vi "CPP_HalveFirstAndLast.vi"(3 "InputArray":dbl[](array[numeric])) -> (1 "HalvedEnds":dbl[](array[numeric]))   [LabVIEW 2010]
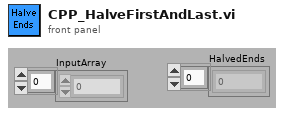
[diagram p1: front panel]
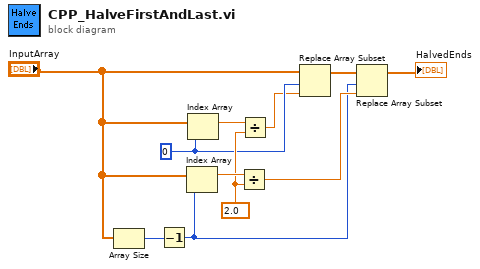
[diagram p0: block diagram]
diagram:
  w7 = 0
  w8 = 2.0
  n1 = Array Size(array="InputArray") -> (size(s)=w3:i32)
  n2 = Decrement(x=w3) -> (x-1=w4:i32)
  n3 = Index Array(array="InputArray", index=w4) -> (element=w9:dbl)
  n4 = Index Array(array="InputArray", index=w7) -> (element=w10:dbl)
  n5 = Divide(x=w9, y=w8) -> (x/y=w5:dbl)
  n6 = Divide(x=w10, y=w8) -> (x/y=w6:dbl)
  n7 = Replace Array Subset(array="InputArray", new element=w6, index=w7) -> (w11:dbl[])
  n8 = Replace Array Subset(array=w11, new element=w5, index=w4) -> (→"HalvedEnds":dbl[])
